vi "Check ESTOP.vi"(8 "error in":errorcluster, 11 "Gantry in":refnum<class "Gantry Class.lvclass">) -> (0 "error out":errorcluster, 3 "Gantry out":refnum<class "Gantry Class.lvclass">)   [LabVIEW 2011, in "Gantry Class.lvclass"]
uses:
  Gantry Class.lvclass
  Gantry Class.lvclass/Gantry Class.ctl
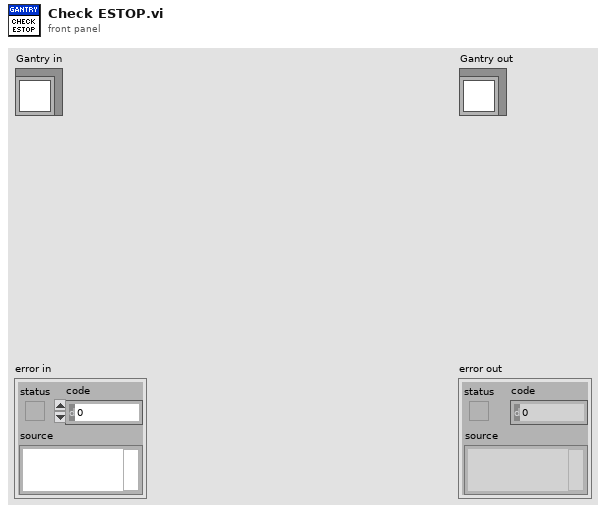
[diagram p1: front panel]
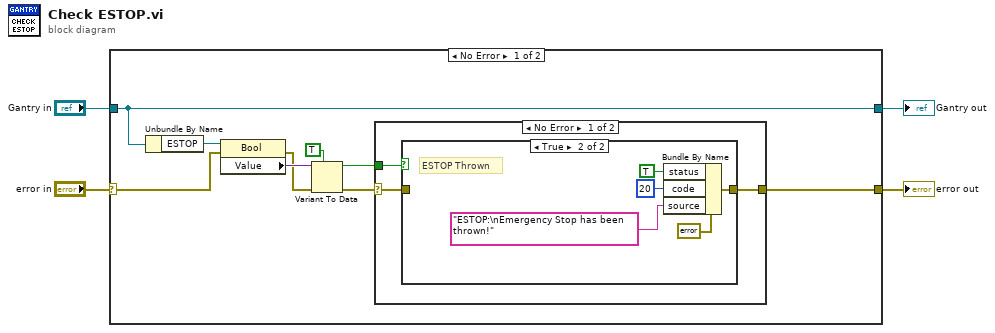
[diagram p0: block diagram]
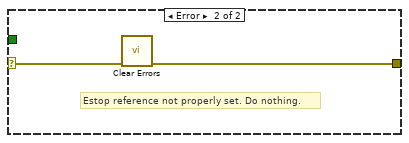
[diagram p3: hidden frame]
diagram:
  n1 = case shown="No Error" "error in" {
    selector: "error in" -> [w5 w26]
    tunnel: [w7 w26] -> w3
    tunnel: [w13 w25] -> w1
    tunnel: "Gantry in" -> [w13 w25]
    frame No Error {
      n2 = Unbundle By Name(w13) -> ("ESTOP"=w6:refnum<vi>)
      n3 = property class="Bool"(reference=w6, error in=w5) -> (error out=w10:errorcluster, "Value"=w12:variant)  [unwired: 1 out]
      n4 = Variant To Data(error in=w10, type=TRUE, Variant=w12) -> (data=w8:bool, error out=w9:errorcluster)
      n5 = case shown="No Error" w9 {
        selector: w9 -> [w15 w24]
        tunnel: w8 -> [w16 _]
        tunnel: [w14 w23] -> w7
        frame No Error {
          n6 = case shown="True" w16 {
            tunnel: w15 -> [w17 _]
            tunnel: [w17 w21] -> w14
            frame False {
            }
            frame True {
              # "ESTOP Thrown"
              n7 = Bundle By Name(cluster=errorcluster {"status"=FALSE, "code"=0, "source"=""} ("error constant"), "status"=TRUE, "code"=20, "source"="ESTOP:\nEmergency Stop has been thrown!") -> (w21:errorcluster)
            }
          }
        }
        frame Error {
          # "Estop reference not properly set. Do nothing."
          n8 = call <vilib>:"Clear Errors.vi"("error in (no error)"=w24) -> ("error out"=w23:errorcluster)  [unwired: 6 in]
        }
      }
    }
    frame Error {
    }
  }
  "error out" <- w3
  "Gantry out" <- w1
